vi "Continuous Graph Update_2.vi"(0 "Bias Voltage":dbl[](array[numeric]), 5 "Resitance":dbl[](array[numeric]), 7 "Stop_V":dbl, 9 "Port 1 Cap":dbl[](array[numeric]), 11 "Port 2 Cap":dbl[](array[numeric])) -> ()   [LabVIEW 2013]
panel:
  out "Error Out":errorcluster
  in  "Error In":errorcluster
  out "Graph Cluster":T1
  in  "error in (no error)":errorcluster
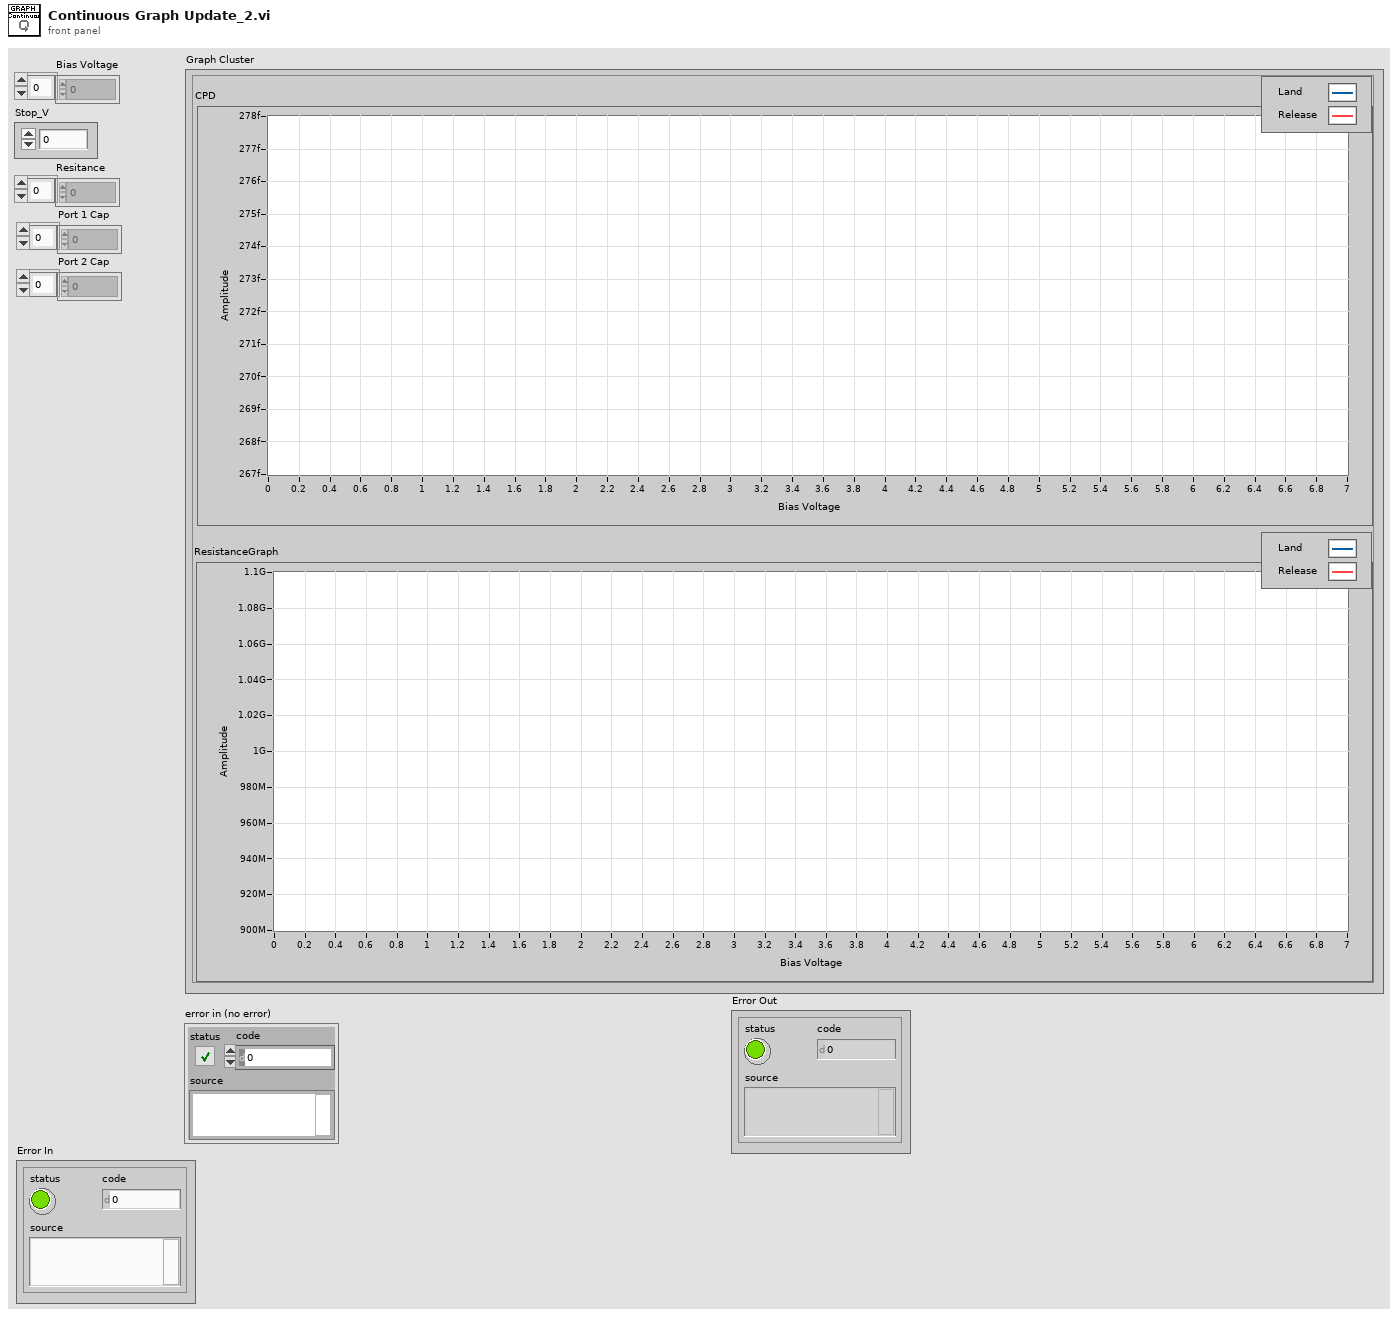
[diagram p1: front panel]
types:
  T1 = cluster{"ResistanceGraph":cluster{dbl[], dbl[]}[], "CPD":cluster{dbl[], dbl[]}[]}
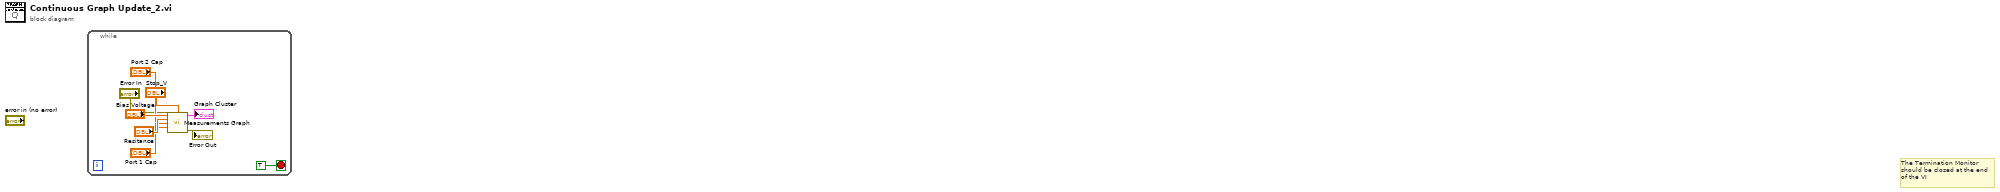
[diagram p0: block diagram]
diagram:
  # "The Termination Monitor\nshould be closed at the end\nof the VI"
  n1 = while {
    stop <- TRUE stop-if-true
    n2 = call "Measurements Graph.vi"("Bias Voltage"="Bias Voltage", "Stop_V"="Stop_V", "Resitance"="Resitance", "Port 1 Cap"="Port 1 Cap", "Port 2 Cap"="Port 2 Cap", "Error In"="Error In") -> ("Graph Cluster"=→"Graph Cluster":T1, "Error Out"=→"Error Out":errorcluster)  [unwired: 8 in]
  }
